vi "NetworkTriggerDAQ_UDP.vi"() -> ()   [LabVIEW 2020]
uses:
  <vilib>/Utility/tcp.llb/UDP Multicast Write-Only Open.vi
panel:
  out "GEECS computer IP":string
  in  "address":string="239.192.5.35"
  in  "receiver port":u16=61000
  in  "ms to add to timestamp":i64=50
  in  "simulate":bool
  out "loop time":u32
  out "error send":errorcluster
  out "error udp open":errorcluster
  out "loop":i32
  out "error daq":errorcluster caption="error out"
  in  "Stop":bool
  in  "device name":tag="Dev2"
  # "this is the wait time in reciever before acquiring"
  # "in PW, run on 15.44"
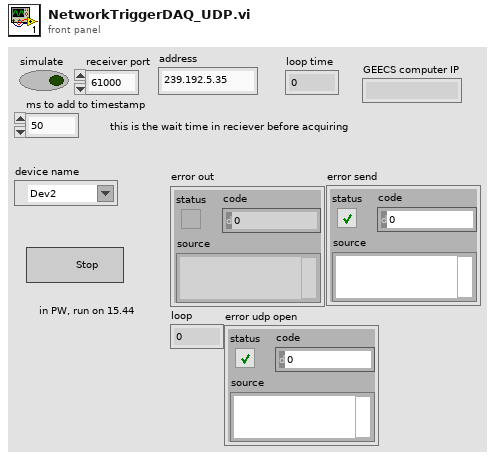
[diagram p1: front panel]
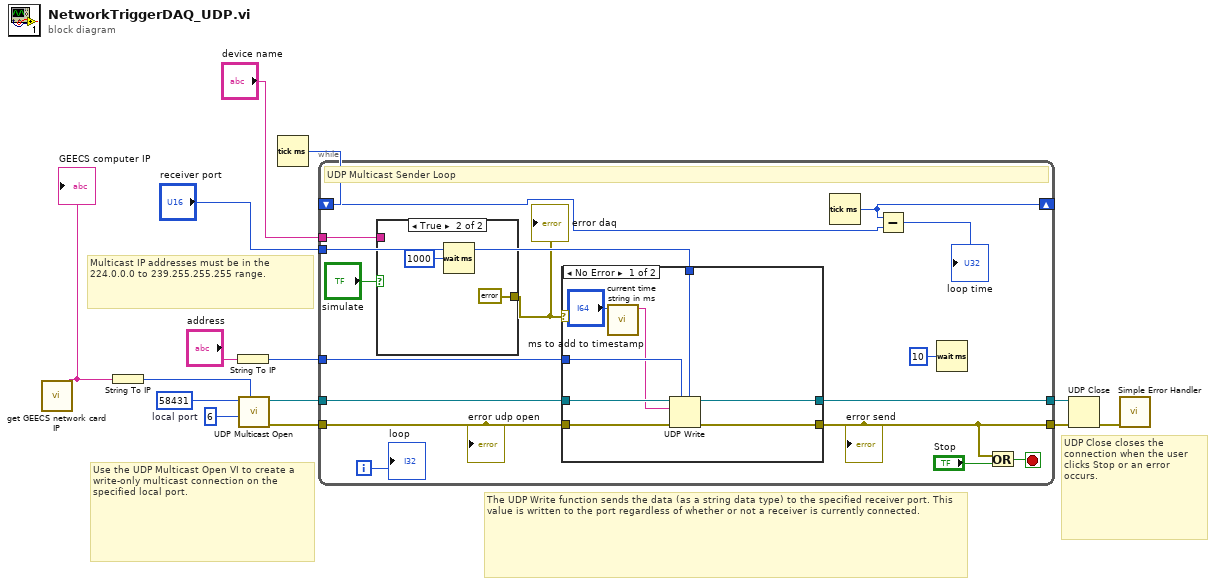
[diagram p0: block diagram]
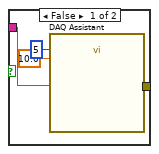
[diagram p2: hidden frame]
diagram:
  w7 = u16 58431  # local port
  # "UDP Close closes the connection when the user clicks Stop or an error occurs."
  # "Multicast IP addresses must be in the 224.0.0.0 to 239.255.255.255 range."
  # "The UDP Write function sends the data (as a string data type) to the specified receiver port. This value is written to the port regardless of whether or not a receiver is currently connected."
  # "Use the UDP Multicast Open VI to create a write-only multicast connection on the specified local port."
  n1 = call "get GEECS network card IP.vi"() -> ("GEECS computer IP"=w2:string)  [unwired: 11 in]
  "GEECS computer IP" <- w2
  n2 = String To IP(1:w2) -> (0:w1:u32)
  n3 = String To IP(1:"address") -> (0:w10:u32)
  n4 = call-poly <vilib>:"UDP Multicast Open.vi"("net address"=w1, "time-to-live (1)"=u16 6, "port"=w7) -> ("error out"=w8:errorcluster, "connection ID"=w9:refnum<k16>)  [unwired: 7 in]
  n5 = Tick Count (ms)() -> (millisecond timer value=w3:u32)
  n6 = while {
    tunnel: [w25] -> w13
    tunnel: w9 -> [w30]
    tunnel: w8 -> [w29]
    tunnel: [w26] -> w14
    tunnel: w10 -> [w24]
    tunnel: "receiver port" -> [w22]
    tunnel: "device name" -> [w21]
    shift-right: [w16] -> _
    shift-left: w3 -> [w18]
    i -> [w19]
    stop <- w28 stop-if-true
    # "UDP Multicast Sender Loop"
    n7 = case shown="True" "simulate" {
      tunnel: w21 -> [w34 _]
      tunnel: [w33 errorcluster {"status"=FALSE, "code"=0, "source"=""} ("error out")] -> w20
      frame False {
        n8 = call "DAQ Assistant"("number of samples"=5, "timeout (s)"=10.0, "device name"=w34) -> ("error out"=w33:errorcluster)  [unwired: 14 in, 2 out]
      }
      frame True {
        n9 = Wait (ms)(milliseconds to wait=u32 1000) -> ()  [unwired: 1 out]
      }
    }
    "error daq" <- w20
    n10 = case shown="No Error" w20 {
      tunnel: w30 -> [w44 w46]
      tunnel: w29 -> [w43 w45]
      tunnel: [w42 w46] -> w26
      tunnel: [w41 w45] -> w25
      tunnel: w24 -> [w40 _]
      tunnel: w22 -> [w39 _]
      frame No Error {
        n11 = call "current time string in ms.vi"("ms to add"="ms to add to timestamp") -> ("time string in ms"=w38:string)  [unwired: 10 in]
        n12 = UDP Write(address=w40, port or service name=w39, connection ID=w44, data in=w38, 8:w43) -> (error out=w41:errorcluster, 3:w42:refnum<k16>)  [unwired: 1 in]
      }
      frame Error {
      }
    }
    "error send" <- w25
    n13 = Tick Count (ms)() -> (millisecond timer value=w16:u32)
    n14 = Subtract(x=w16, y=w18) -> (x-y=→"loop time":u32)
    n15 = Wait (ms)(milliseconds to wait=u32 10) -> ()  [unwired: 1 out]
    n16 = Or(x=w25, y="Stop") -> (x .or. y?=w28:bool)
    "loop" <- w19
    "error udp open" <- w29
  }
  n17 = UDP Close(connection ID=w14, 8:w13) -> (error out=w11:errorcluster)  [unwired: 1 out]
  n18 = call <vilib>:"Simple Error Handler.vi"("error in (no error)"=w11) -> ()  [unwired: 4 in, 5 out]
